vi "Get CD Item Property Value.vi"(8 "error in (no error)":errorcluster, 10 "CD Item Ref in":T1 format="%.0x", 11 "Double Parameter in":refnum<class "Double Parameter.lvclass">) -> (0 "error out":errorcluster, 3 "Double Parameter out":refnum<class "Double Parameter.lvclass">)   [LabVIEW 2019, in "CD Parameter Manager API.lvlib" / "Double Parameter.lvclass"]
uses:
  Double Parameter.lvclass
  C:/Repositories/UI-Control-Initializer-API/Source/Parameter Class/Parameter.lvclass
  <vilib>/NI VeriStand/Custom Device API/Custom Device Item Ref.ctl
  Parameter Class/Parameter.lvclass/Parameter.ctl
  Double Parameter.lvclass/Double Parameter.ctl
  Parameter Class/Member Accessors/Read Control label.vi
  Member Accessors/Read Value.vi
  Member Accessors/Write Value.vi
  <vilib>/NI VeriStand/Custom Device API/Get Item Property (Double).vi
  <vilib>/NI VeriStand/Custom Device API/Custom Device API.lvlib
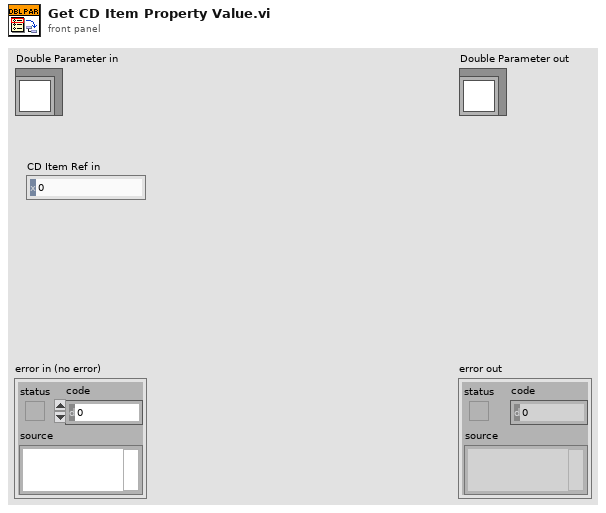
[diagram p1: front panel]
types:
  T1 = typedef "Custom Device API.lvlib/Custom Device Item Ref.ctl" = u64
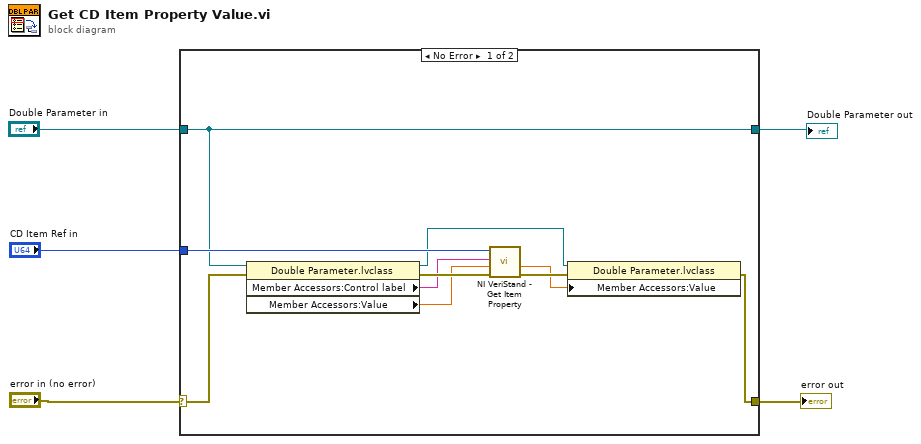
[diagram p0: block diagram]
diagram:
  n1 = case shown="No Error" "error in (no error)" {
    selector: "error in (no error)" -> [w14 w16]
    tunnel: [w8 w16] -> w4
    tunnel: "CD Item Ref in" -> [w15 _]
    tunnel: [w13 w17] -> w5
    tunnel: "Double Parameter in" -> [w13 w17]
    frame No Error {
      n2 = property class="Double Parameter.lvclass"(reference=w13, error in=w14) -> (reference out=w6:refnum<class "Double Parameter.lvclass">, error out=w12:errorcluster, "Member Accessors:Control label"=w11:string, "Member Accessors:Value"=w10:dbl)
      n3 = call-poly <vilib>:"NI VeriStand - Get Item Property.vi"("error in (no error)"=w12, "Default Value"=w10, "Property Name"=w11, "Item Ref in"=w15) -> ("error out"=w9:errorcluster, "Value"=w7:dbl)  [unwired: 4 in, 2 out]
      n4 = property class="Double Parameter.lvclass"(reference=w6, error in=w9, "Member Accessors:Value"=w7) -> (error out=w8:errorcluster)  [unwired: 1 out]
    }
    frame Error {
    }
  }
  "error out" <- w4
  "Double Parameter out" <- w5
